vi "FieldDisp_Field_Disp.vi"(5 "Field X Ft":dbl=58.0 format="%#_13g", 7 "Field Y Ft":dbl=27.0 format="%#_13g", 9 "Field Selector":string, 11 "Picture in":refnum<vi>) -> (0 "error out":errorcluster)   [LabVIEW 2019, in "Trajectory_Library.lvlib"]
doc: "Read the specified field image file, scale and crop the image, then update the picture control with the image.\n\nThe field information INI file must be in a FieldInfo subdirectory under the application's main directory. The field image files are also located in this subdirectory.\n\nInputs:\n - Picture In -- Picture Control Reference -- Reference to the picture control to display the field..\n - Field Selector -- String -- String containing the name of the field to display. This can be the output of a combo box control.\n\nOutputs:\n - Error out -- error cluster -- If an error occured, contains error information."
uses:
  Trajectory_Library.lvlib
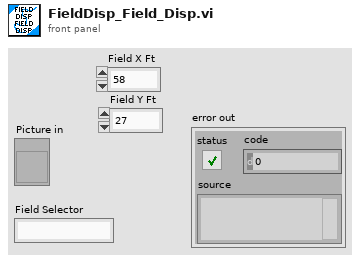
[diagram p1: front panel]
types:
  T1 = typedef "Trajectory_Library.lvlib/FieldDisp_Field_Info.ctl" = cluster{"FIeld_File_Name":string, "Top_Left_X_Pix":i32, "Top_Left_Y_Pix":i32, "Bottom_Right_X_Pix":i32, "Bottom_Right_Y_Pix":i32, "Field_Size_X_Ft":dbl, "Field_Size_Y_Ft":dbl, "FIeld_Size_Units":string}
  T2 = typedef "IMAQ Image.ctl" = refnum<image>
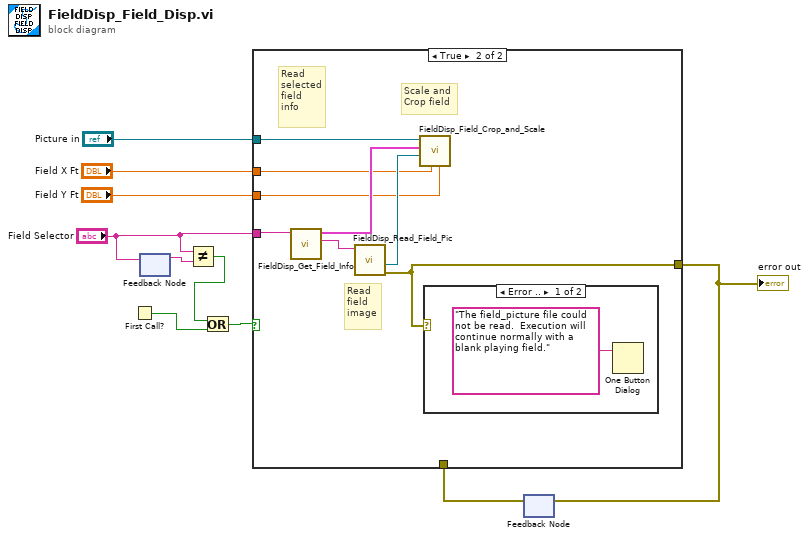
[diagram p0: block diagram]
diagram:
  n1 = First Call?() -> (First Call?: T/F=w8:bool)
  n2 = feedback #1() -> (w6:string)  [unwired: 1 in]
  n3 = feedback-in #1("Field Selector") -> ()
  n4 = Not Equal?(x="Field Selector", y=w6) -> (x != y?=w9:bool)
  n5 = Or(x=w9, y=w8) -> (x .or. y?=w7:bool)
  n6 = feedback #2() -> (w3:errorcluster)  [unwired: 1 in]
  n7 = case shown="True" w7 {
    tunnel: "Field Selector" -> [_ w17]
    tunnel: "Picture in" -> [_ w16]
    tunnel: [w11 w14] -> w4
    tunnel: w3 -> [w11 _]
    tunnel: "Field X Ft" -> [_ w13]
    tunnel: "Field Y Ft" -> [_ w12]
    frame False {
    }
    frame True {
      # "Scale and\nCrop field"
      # "Read\nfield\nimage"
      # "Read\nselected\nfield\ninfo"
      n8 = call "FieldDisp_Get_Field_Info.vi"("Field Selector"=w17) -> ("File"=w19:string, "Field Info"=w18:T1)  [unwired: 9 in]
      n9 = call "FieldDisp_Read_Field_Pic.vi"("file name"=w19) -> ("Image Error"=w14:errorcluster, "Image Out"=w15:T2)  [unwired: 7 in, 2 out]
      n10 = call "FieldDisp_Field_Crop_and_Scale.vi"("Field Y Ft"=w12, "Field X Ft"=w13, "Field Image"=w15, "field Info"=w18, "Field Picture Ref"=w16) -> ()  [unwired: 6 in, 1 out]
      n11 = case shown="Error .." w14 {
        frame Error {
          n12 = One Button Dialog(message="The field_picture file could not be read.  Execution will continue normally with a blank playing field.") -> ()  [unwired: 1 in, 1 out]
        }
        frame No Error {
        }
      }
    }
  }
  "error out" <- w4
  n13 = feedback-in #2(w4) -> ()
